vi "Status.vi"(8 "error in (no error)":errorcluster, 10 "Internal?":bool, 11 "Julabo FP-50 Settings In":T1={"VISA resource name"="", "Simulated?"=FALSE, "Pump Power"=2} {"Pump Power" min=0 max=8 step=1}) -> (0 "error out":errorcluster, 1 "Connection Error":bool, 2 "Running":bool, 3 "Julabo FP-50 Settings Out":T1={"VISA resource name"="", "Simulated?"=FALSE, "Pump Power"=2} {"Pump Power" min=0 max=8 step=1}, 4 "Temp":dbl, 6 "Pumpstage (out)":u8)   [LabVIEW 2021, in "Julabo Type FP-50 TCU.lvlib"]
uses:
  Julabo Type FP-50 TCU.lvlib
  Julabo FP-50 Settings.ctl
  Third Party Drivers/Julabo Type 1/JULABO DeviceDriver/JULABO DeviceDriver.lvlib
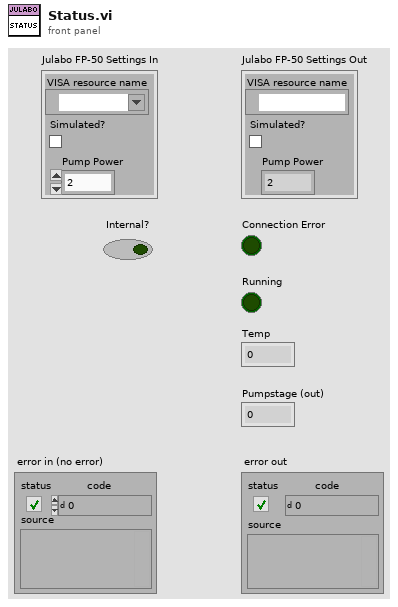
[diagram p1: front panel]
types:
  T1 = typedef "Julabo Type FP-50 TCU.lvlib/Julabo FP-50 Settings.ctl" = cluster{"VISA resource name":refnum<visa-resource-name>, "Simulated?":bool, "Pump Power":i32}
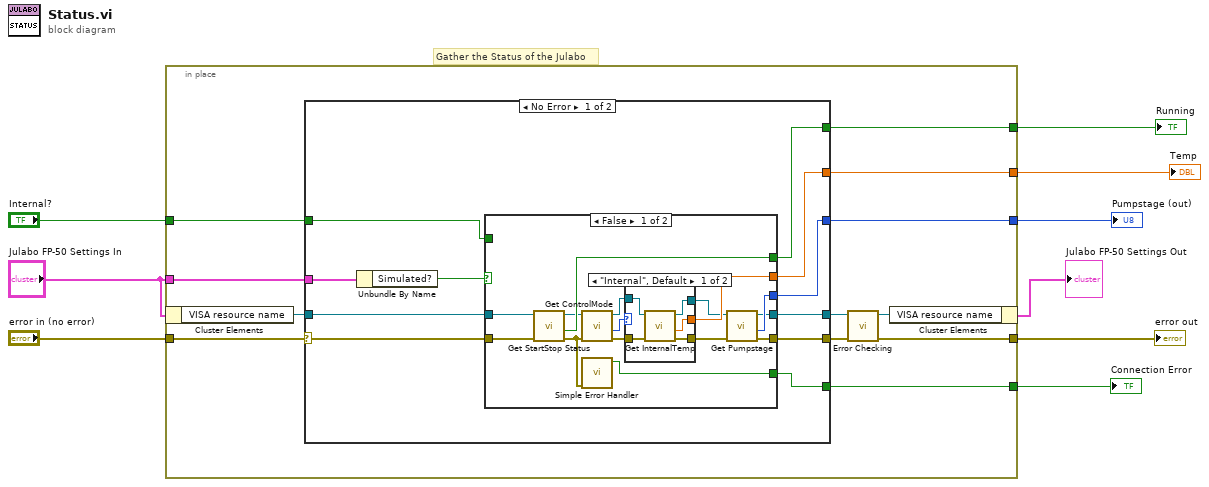
[diagram p0: block diagram]
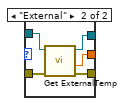
[diagram p2: hidden frame]
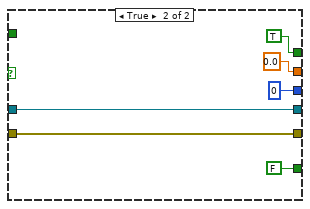
[diagram p3: hidden frame]
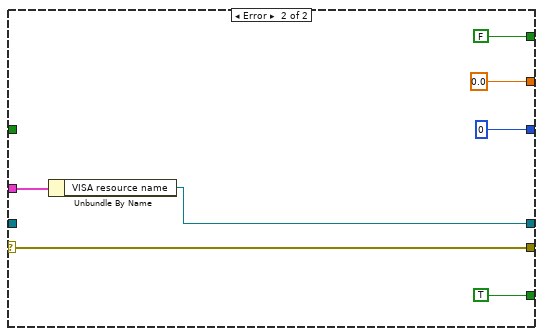
[diagram p4: hidden frame]
diagram:
  # "Gather the Status of the Julabo"
  n1 = in-place {
    in-place-border: "error in (no error)" -> [w21]
    in-place-border: [w18] -> w8
    in-place-border: "Julabo FP-50 Settings In" -> [w17]
    in-place-border: [w16] -> w7
    in-place-border: [w15] -> w6
    in-place-border: "Internal?" -> [w14]
    in-place-border: [w13] -> w4
    in-place-border: [w12] -> w3
    n2 = in-place-cluster #1("Julabo FP-50 Settings In") -> ("VISA resource name"=w11:refnum<visa-resource-name>)
    n3 = case shown="No Error" w21 {
      selector: w21 -> [w32 w70]
      tunnel: w17 -> [w30 w69]
      tunnel: [w31 w70] -> w19
      tunnel: [w29 w68] -> w20
      tunnel: [w27 TRUE] -> w16
      tunnel: [w26 FALSE] -> w15
      tunnel: w14 -> [w25 _]
      tunnel: [w24 0.0 ("InternalTemp (out)")] -> w13
      tunnel: [w23 u8 0 ("Pumpstage (out)")] -> w12
      tunnel: w11 -> [w22 _]
      frame No Error {
        n4 = Unbundle By Name(w30) -> ("Simulated?"=w28:bool)
        n5 = case shown="False" w28 {
          tunnel: w32 -> [w46 w63]
          tunnel: [w33 w63] -> w31
          tunnel: [w35 w62] -> w29
          tunnel: w22 -> [w47 w62]
          tunnel: [w44 FALSE] -> w27
          tunnel: [w45 TRUE] -> w26
          tunnel: w25 -> [_ _]
          tunnel: [w43 0.0 ("InternalTemp (out)")] -> w24
          tunnel: [w37 u8 0 ("Pumpstage (out)")] -> w23
          frame False {
            n6 = call "Get StartStop Status.vi"("error in"=w46, "VISA resource name in"=w47) -> ("error out"=w41:errorcluster, "Status"=w45:bool, "VISA resource name out"=w42:refnum<visa-resource-name>)  [unwired: 7 in]
            n7 = call "Get ControlMode.vi"("error in"=w41, "VISA resource name in"=w42) -> ("error out"=w38:errorcluster, "Control (out)"=w40:enum16{"Internal", "External"}, "VISA resource name out"=w39:refnum<visa-resource-name>)  [unwired: 7 in]
            n8 = call <vilib>:"Simple Error Handler.vi"("error in (no error)"=w41) -> ("error?"=w44:bool)  [unwired: 4 in, 4 out]
            n9 = case shown="\"Internal\", Default" w40 {
              tunnel: w39 -> [w52 w57]
              tunnel: w38 -> [w51 w56]
              tunnel: [w50 w54] -> w36
              tunnel: [w49 w55] -> w34
              tunnel: [w48 w53] -> w43
              frame "Internal", Default {
                n10 = call "Get InternalTemp.vi"("error in (no error)"=w51, "VISA resource name"=w52) -> ("error out"=w49:errorcluster, "InternalTemp (out)"=w48:dbl, "VISA resource name out"=w50:refnum<visa-resource-name>)  [unwired: 7 in]
              }
              frame "External" {
                n11 = call "Get ExternalTemp.vi"("error in (no error)"=w56, "VISA resource name"=w57) -> ("error out"=w55:errorcluster, "ExternalTemp (out)"=w53:dbl, "VISA resource name out"=w54:refnum<visa-resource-name>)  [unwired: 6 in, 1 out]
              }
            }
            n12 = call "Get Pumpstage.vi"("error in (no error)"=w34, "VISA resource name"=w36) -> ("error out"=w33:errorcluster, "Pumpstage (out)"=w37:u8, "VISA resource name out"=w35:refnum<visa-resource-name>)  [unwired: 7 in]
          }
          frame True {
          }
        }
      }
      frame Error {
        n13 = Unbundle By Name(w69) -> ("VISA resource name"=w68:refnum<visa-resource-name>)
      }
    }
    n14 = call "Error Checking.vi"("error in (no error)"=w19, "VISA resource name"=w20) -> ("error out"=w18:errorcluster, "VISA resource name"=w10:refnum<visa-resource-name>)  [unwired: 7 in, 1 out]
    n15 = in-place-cluster #1("VISA resource name"=w10) -> (→"Julabo FP-50 Settings Out":T1)
  }
  "error out" <- w8
  "Connection Error" <- w7
  "Running" <- w6
  "Temp" <- w4
  "Pumpstage (out)" <- w3
